vi "Calculate Normal Array.vi"(8 "error in (no error)":errorcluster, 9 "Coordinates System":enum16{"Cartesian", "Cylindrical", "Spherical"}(ring), 10 "3D Contour Datatype.lvclass in":refnum<class "3D Contour Datatype.lvclass">, 11 "Plot Representation In":T1) -> (0 "error out":errorcluster, 1 "Dup Coordinates System":enum16{"Cartesian", "Cylindrical", "Spherical"}(ring), 2 "3D Contour Datatype.lvclass out":refnum<class "3D Contour Datatype.lvclass">, 3 "Plot Representation Out":T1)   [LabVIEW 2020, in "3D Contour Datatype.lvclass"]
uses:
  <vilib>/Math Plots/3D Math Plots/3D Contour/3D Contour Datatype/3D Contour Datatype.lvclass
  <vilib>/Math Plots/3D Math Plots/3D Plot/3D Plot/Typedef/Plot Representation.ctl
  <vilib>/Math Plots/3D Math Plots/3D Plot/3D Plot/Typedef/Range Clusters.ctl
  <vilib>/Math Plots/3D Math Plots/3D Plot/3D Plot/Typedef/Mesh Data.ctl
  <vilib>/Math Plots/3D Math Plots/3D Plot/3D Plot Datatype/3D Plot Datatype.lvclass
  <vilib>/Math Plots/3D Math Plots/3D Plot/3D Plot/3D Plot.lvclass
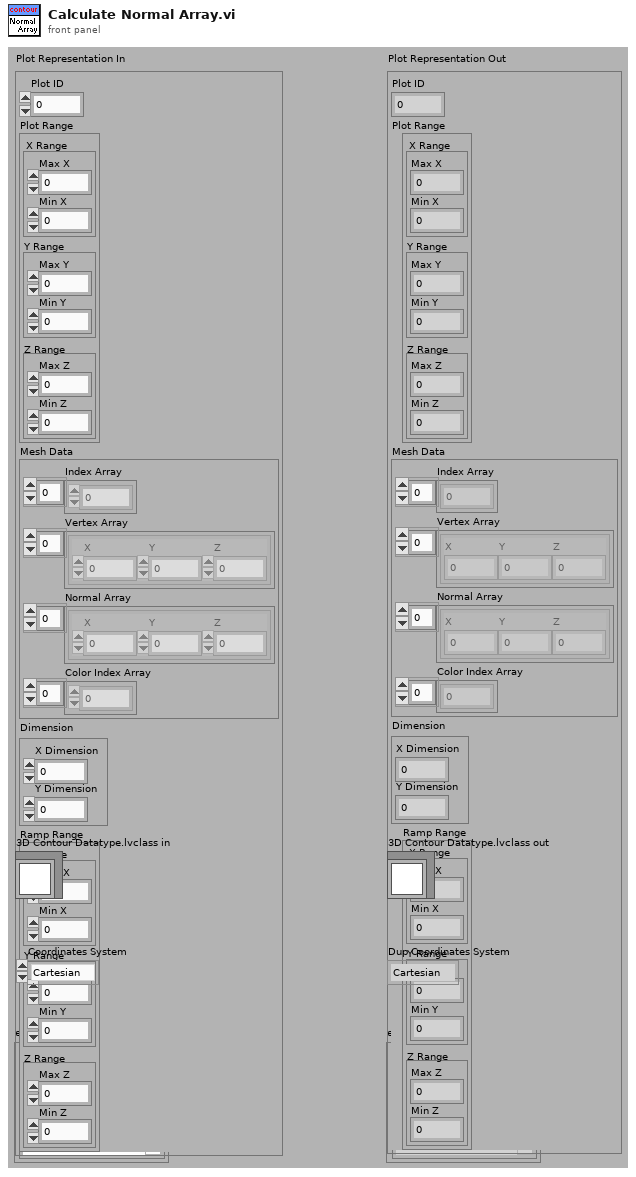
[diagram p1: front panel]
types:
  T1 = typedef "3D Plot.lvclass/Plot Representation.ctl" = cluster{"Plot ID":i32, "Plot Range":T2, "Mesh Data":T3, "Dimension":cluster{"X Dimension":i32, "Y Dimension":i32}, "Ramp Range":T2}
  T2 = typedef "3D Plot.lvclass/Range Clusters.ctl" = cluster{"X Range":cluster{"Max X":sgl, "Min X":sgl}, "Y Range":cluster{"Max Y":sgl, "Min Y":sgl}, "Z Range":cluster{"Max Z":sgl, "Min Z":sgl}}
  T3 = typedef "3D Plot.lvclass/Mesh Data.ctl" = cluster{"Index Array":u32[], "Vertex Array":cluster{"X":sgl, "Y":sgl, "Z":sgl}[], "Normal Array":cluster{"X":sgl, "Y":sgl, "Z":sgl}[], "Color Index Array":i32[]}
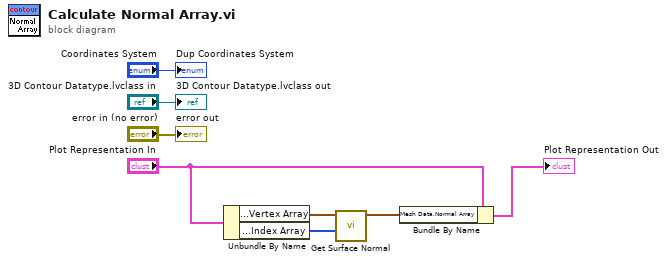
[diagram p0: block diagram]
diagram:
  n1 = Unbundle By Name("Plot Representation In") -> ("Mesh Data.Vertex Array"=w3:cluster{"X":sgl, "Y":sgl, "Z":sgl}[], "Mesh Data.Index Array"=w1:u32[])
  n2 = call <vilib>:"Get Surface Normal.vi"("Triangle Index Array"=w1, "Vertex Array"=w3) -> ("Normal Array"=w2:cluster{"X":sgl, "Y":sgl, "Z":sgl}[])  [unwired: 9 out]
  n3 = Bundle By Name(cluster="Plot Representation In", "Mesh Data.Normal Array"=w2) -> (→"Plot Representation Out":T1)
  "error out" <- "error in (no error)"
  "3D Contour Datatype.lvclass out" <- "3D Contour Datatype.lvclass in"
  "Dup Coordinates System" <- "Coordinates System"
